vi "Set Inline Buffer.vi"(8 "error in (no error)":errorcluster, 10 "command parameters":T1, 11 "Plugin Thread in":refnum<class "Plugin Thread.lvclass">) -> (0 "error out":errorcluster, 3 "Plugin Thread out":refnum<class "Plugin Thread.lvclass">)   [LabVIEW 2017, in "DSF Core.lvlib" / "Plugin Thread.lvclass"]
uses:
  Thread/Plugin/Plugin Thread.lvclass
  Interfaces/Plugin/Command Parameters.ctl
  Interfaces/Plugin/Response Data.ctl
  Interfaces/Plugin/Response.ctl
  Interfaces/Plugin/Response Parameters.ctl
  Buffer/Buffer.lvclass
  C:/Program Files (x86)/National Instruments/LabVIEW 2017/vi.lib/NI/Memory Manager/Classes/Pointer/Pointer.lvclass
  Thread/Plugin/Plugin Thread.lvclass/Plugin Thread.ctl
  <vilib>/NI/Memory Manager/Classes/Pointer/Pointer.lvclass/Pointer.ctl
  <vilib>/NI/Memory Manager/Classes/Pointer/Set Size.vi
  <vilib>/NI/Memory Manager/Classes/Pointer/Set Address.vi
  <vilib>/NI/Memory Manager/Classes/Pointer/Check Null Pointer.vi
  <vilib>/NI/Memory Manager/Classes/Pointer/Set Internal.vi
  <vilib>/NI/Memory Manager/Classes/Pointer/Errors.vi
  <vilib>/NI/Memory Manager/Classes/Pointer/Null Pointer.vi
  <vilib>/NI/Memory Manager/Classes/Pointer/Is Null.vi
  <vilib>/NI/Memory Manager/Classes/Pointer/Create Error.vi
  <vilib>/NI/Memory Manager/Classes/Pointer/Get Address.vi
  <vilib>/NI/Memory Manager/VIs/New Error Cluster Constant.vi
  <vilib>/NI/Memory Manager/VIs/New Error Cluster Constant (512B).vi
  <vilib>/NI/Memory Manager/VIs/Error Cluster.Set Status.vi
  <vilib>/NI/Memory Manager/VIs/Error Cluster.Set Code.vi
  <vilib>/NI/Memory Manager/VIs/Error Cluster.Set VI Source.vi
  <vilib>/NI/Memory Manager/Constants/Constants.vi
  <vilib>/NI/Memory Manager/Constants/Library Name.vi
  <vilib>/NI/Memory Manager/Classes/Pointer/Pointer Error Info.vi
  <vilib>/NI/Memory Manager/VIs/Source.Write.String.vi
  <vilib>/NI/Memory Manager/Constants/Pointer Class Name.vi
  Interfaces/Plugin/Plugin Interface.lvclass
  <vilib>/NI/Memory Manager/Classes/Pointer/Pointer.lvclass
  Transfer Group/Transfer Group.lvclass
  Buffer/Buffers.lvclass
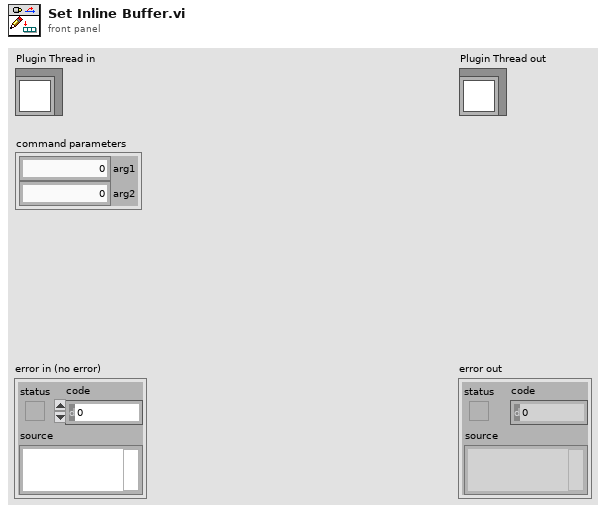
[diagram p1: front panel]
types:
  T1 = typedef "DSF Core.lvlib/Plugin Interface.lvclass/Command Parameters.ctl" = cluster{"arg1":u64, "arg2":u64}
  T2 = typedef "DSF Core.lvlib/Plugin Interface.lvclass/Response Data.ctl" = cluster{"Response":T3, "Parameters":T4}
  T3 = typedef "DSF Core.lvlib/Plugin Interface.lvclass/Response.ctl" = enum8{"General Ack", "Shutting Down"}
  T4 = typedef "DSF Core.lvlib/Plugin Interface.lvclass/Response Parameters.ctl" = cluster{"arg1":u64, "arg2":u64}
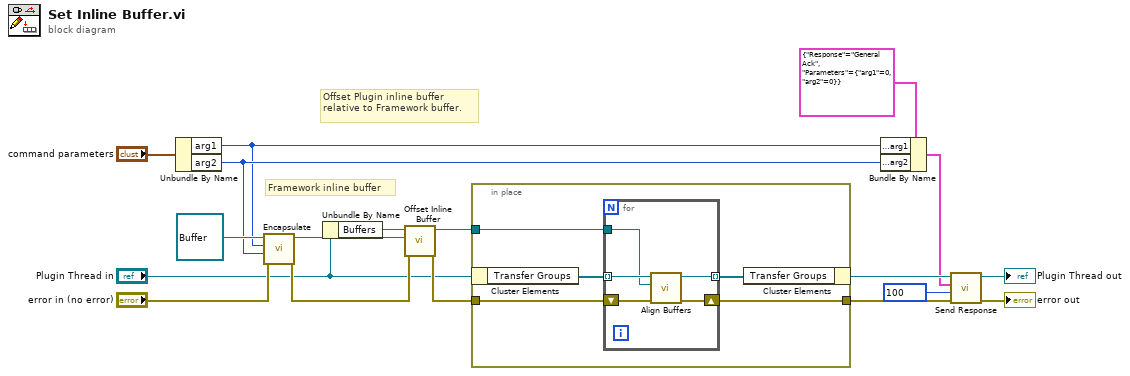
[diagram p0: block diagram]
diagram:
  # "Offset Plugin inline buffer relative to Framework buffer."
  # "Framework inline buffer"
  n1 = Unbundle By Name("command parameters") -> ("arg1"=w1:u64, "arg2"=w2:u64)
  n2 = call <vilib>:"Encapsulate.vi"("error in (no error)"="error in (no error)", "size"=w2, "address"=w1, "Pointer in"=refnum<class "Buffer.lvclass"> refnum ("base Buffer")) -> ("error out"=w8:errorcluster, "Pointer out"=w5:refnum<class "Buffer.lvclass">)  [unwired: 6 in]
  n3 = Unbundle By Name("Plugin Thread in") -> ("Buffers"=w3:refnum<class "Buffers.lvclass">)
  n4 = call "Offset Inline Buffer.vi"("error in (no error)"=w8, "base Inline Buffer"=w5, "Buffers in"=w3) -> ("error out"=w7:errorcluster, "Buffers out"=w9:refnum<class "Buffers.lvclass">)  [unwired: 7 in]
  n5 = in-place {
    in-place-border: [w21] -> w13
    in-place-border: w7 -> [w20]
    in-place-border: w9 -> [w19]
    n6 = in-place-cluster #1("Plugin Thread in") -> ("Transfer Groups"=w23:refnum<class "Transfer Group.lvclass">[])
    n7 = for {
      tunnel: w23 -> [w28] mode=indexing
      tunnel: [w27] -> w22 mode=indexing
      shift-right: [w26] -> w21
      shift-left: w20 -> [w25]
      tunnel: w19 -> [w24]
      n8 = call "Align Buffers.vi"("error in (no error)"=w25, "Plugin Buffers"=w24, "Transfer Group in"=w28) -> ("error out"=w26:errorcluster, "Transfer Group out"=w27:refnum<class "Transfer Group.lvclass">)  [unwired: 7 in]
    }
    n9 = in-place-cluster #1("Transfer Groups"=w22) -> (w12:refnum<class "Plugin Thread.lvclass">)
  }
  n10 = Bundle By Name(cluster=T2 {"Response"=enum."General Ack", "Parameters"={"arg1"=0, "arg2"=0}} ("response"), "Parameters.arg1"=w1, "Parameters.arg2"=w2) -> (w10:T2)
  n11 = call "Send Response.vi"("error in (no error)"=w13, "timeout in ms (0)"=100, "response"=w10, "Plugin Thread in"=w12) -> ("error out"=→"error out":errorcluster, "Plugin Thread out"=→"Plugin Thread out":refnum<class "Plugin Thread.lvclass">)  [unwired: 6 in]
